vi "BX.Facade__LCR.vi"(0 "Data In":T11, 2 "Display State In":T2={"Orientation"=0, "ActivePicture"={"image type"=0, "image depth"=0, "image"=[], "mask"=[], "colors"=[], "Rectangle"={"left"=0, "top"=0, "right"=0, "bottom"=0}}, "Pictures"={"Normal"={"image type"=0, "image depth"=0, "image"=[], "mask"=[], "colors"=[], "Rectangle"={"left"=0, "top"=0, "right"=0, "bottom"=0}}, "Hilite"={"image type"=0, "image depth"=0, "image"=[], "mask"=[], "colors"=[], "Rectangle"={"left"=0, "top"=0, "right"=0, "bottom"=0}}}, "Text"={"String"="", "Font"={"Font Name:"="", "Size"=0, "Strikeout?"=FALSE, "Italic?"=FALSE, "Underline?"=FALSE, "Outline?"=FALSE, "Shadow?"=FALSE, "Bold?"=FALSE}, "TextColor"=0}, "RunTimeSettings"={"Highlight"=FALSE, "ShowButton"=FALSE, "Behaviour"=enum."Switch when pressed", "React if disabled"=FALSE, "Nudge Button"=TRUE, "ShowButton on Hover"=FALSE, "Button Type"=enum."System"}, "Messages"=[], "Status"=0, "XControl Label"="", "Boolean Value"=FALSE} {"Status" format="%.0x"}, 3 "Container State":T10) -> (6 "Data Out":T11, 7 "Display State Out":T2={"Orientation"=0, "ActivePicture"={"image type"=0, "image depth"=0, "image"=[], "mask"=[], "colors"=[], "Rectangle"={"left"=0, "top"=0, "right"=0, "bottom"=0}}, "Pictures"={"Normal"={"image type"=0, "image depth"=0, "image"=[], "mask"=[], "colors"=[], "Rectangle"={"left"=0, "top"=0, "right"=0, "bottom"=0}}, "Hilite"={"image type"=0, "image depth"=0, "image"=[], "mask"=[], "colors"=[], "Rectangle"={"left"=0, "top"=0, "right"=0, "bottom"=0}}}, "Text"={"String"="", "Font"={"Font Name:"="", "Size"=0, "Strikeout?"=FALSE, "Italic?"=FALSE, "Underline?"=FALSE, "Outline?"=FALSE, "Shadow?"=FALSE, "Bold?"=FALSE}, "TextColor"=0}, "RunTimeSettings"={"Highlight"=FALSE, "ShowButton"=FALSE, "Behaviour"=enum."Switch when pressed", "React if disabled"=FALSE, "Nudge Button"=TRUE, "ShowButton on Hover"=FALSE, "Button Type"=enum."System"}, "Messages"=[], "Status"=0, "XControl Label"="", "Boolean Value"=FALSE} {"Status" format="%.0x"}, 8 "Action":T1)   [LabVIEW 2011, in "BooleanXControl__LCR.xctl"]
doc: "Facade VI of the XControl"
uses:
  BooleanXControl__LCR.xctl
  BX.Data__LCR.ctl
  <vilib>/_xctls/Container State.ctl
  BX.State__LCR.ctl
  Controls/BX.Orientation__LCR.ctl
  <vilib>/picture/picture.llb/imagedata.ctl
  Controls/BX.RTSettings__LCR.ctl
  Controls/BX.Behaviour__LCR.ctl
  Controls/BX.ButtonType__LCR.ctl
  Controls/BX.Message__LCR.ctl
  Controls/BX.Commands__LCR.ctl
  <vilib>/_xctls/Action.ctl
  Controls/BX.Refs__LCR.ctl
  <userlib>/_OpenG.lib/file/file.llb/Strip Path Extension - Path__ogtk.vi
  <vilib>/Utility/inputDevices.llb/mouseAcquire.vi
  <vilib>/Utility/cursorutil.llb/Set Cursor (Icon Pict).vi
  <vilib>/_xctls/XControlSupport.lvlib
panel:
  in  "HiddenPath":path
  out "BooleanPicture":picture
  in  "ClassicButton":bool
  in  "ModernButton":bool
  out "BooleanString":string
  in  "SystemButton":bool
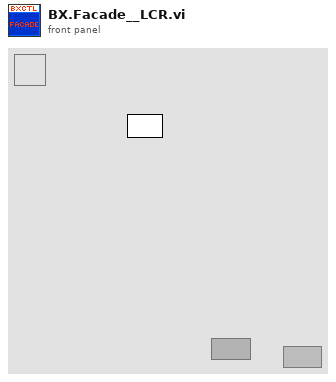
[diagram p1: front panel]
types:
  T1 = typedef "XControlSupport.lvlib/Action.ctl" = cluster{"Data Changed?":bool, "State Changed?":bool, "Action Name":string}
  T2 = typedef "BooleanXControl__LCR.xctl/BX.State__LCR.ctl" = cluster{"Orientation":T3, "ActivePicture":T4, "Pictures":cluster{"Normal":T4, "Hilite":T4}, "Text":cluster{"String":string, "Font":cluster{"Font Name:":string, "Size":i16, "Strikeout?":bool, "Italic?":bool, "Underline?":bool, "Outline?":bool, "Shadow?":bool, "Bold?":bool}, "TextColor":u32}, "RunTimeSettings":T5, "Messages":T8[], "Status":u16, "XControl Label":string, "Boolean Value":bool}
  T3 = typedef "BooleanXControl__LCR.xctl/BX.Orientation__LCR.ctl" = u8
  T4 = typedef "imagedata.ctl" = cluster{"image type":i32, "image depth":i32, "image":u8[], "mask":u8[], "colors":u32[], "Rectangle":cluster{"left":i16, "top":i16, "right":i16, "bottom":i16}}
  T5 = typedef "BooleanXControl__LCR.xctl/BX.RTSettings__LCR.ctl" = cluster{"Highlight":bool, "ShowButton":bool, "Behaviour":T6, "React if disabled":bool, "Nudge Button":bool, "ShowButton on Hover":bool, "Button Type":T7}
  T6 = typedef "BooleanXControl__LCR.xctl/BX.Behaviour__LCR.ctl" = enum16{"Switch when pressed", "Switch when released", "Switch until released"}
  T7 = typedef "BooleanXControl__LCR.xctl/BX.ButtonType__LCR.ctl" = enum16{"System", "Modern", "Classic", "Decoration"}
  T8 = typedef "BooleanXControl__LCR.xctl/BX.Message__LCR.ctl" = cluster{"Command":T9, "Parameter":variant}
  T9 = typedef "BooleanXControl__LCR.xctl/BX.Commands__LCR.ctl" = enum16{"None", "SetPicture", "SetFont", "SetText", "SetOrientation", "Redraw", "SetTextColor", "SetRTSettings", "MultipleUpdate", "RT.Button", "RT.Hilite", "RT.Behaviour", "RT.Disabled", "ShowGUI", "RT.Nudge", "RT.Hover", "RT.ButtonType"}
  T10 = typedef "XControlSupport.lvlib/Container State.ctl" = cluster{"Indicator?":bool, "Run Mode?":bool, " Refnum":refnum<vi>}
  T11 = typedef "BooleanXControl__LCR.xctl/BX.Data__LCR.ctl" = bool
  T12 = typedef "BooleanXControl__LCR.xctl/BX.Refs__LCR.ctl" = cluster{"HiddenPath":refnum<vi>, "String":refnum<vi>, "Picture":refnum<vi>, "XControl":refnum<vi>, "SystemButton":refnum<vi>, "ModernButton":refnum<vi>, "ClassicButton":refnum<vi>, "Decor Refnum":refnum<vi>}
  T13 = cluster{"button 1":bool, "button 2":bool, "button 3":bool, "button 4":bool}
  T14 = typedef "eventsource.ctl" = u32
  T15 = cluster{"Shift":bool, "Ctrl":bool, "Alt":bool, "Cmd":bool, "Opt":bool}
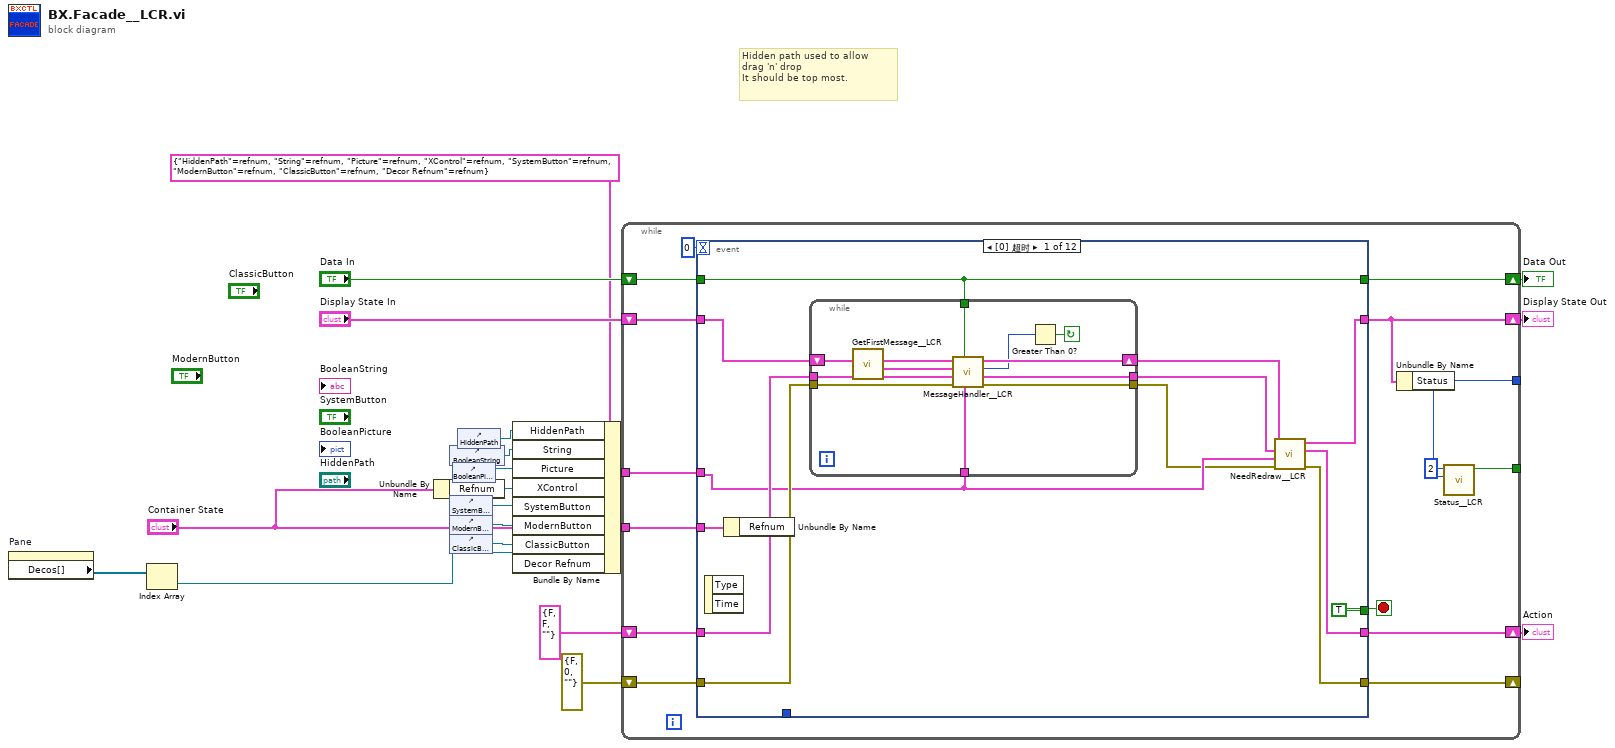
[diagram p0: block diagram]
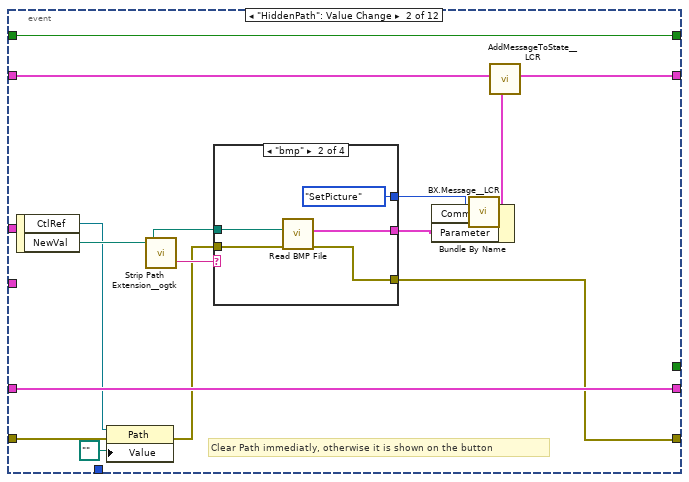
[diagram p2: hidden frame]
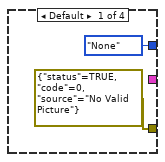
[diagram p3: hidden frame]
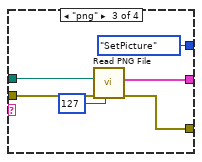
[diagram p4: hidden frame]
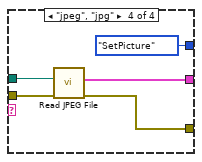
[diagram p5: hidden frame]
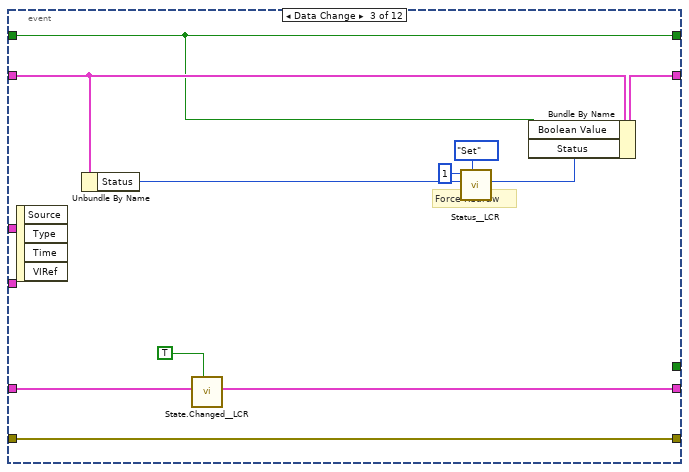
[diagram p6: hidden frame]
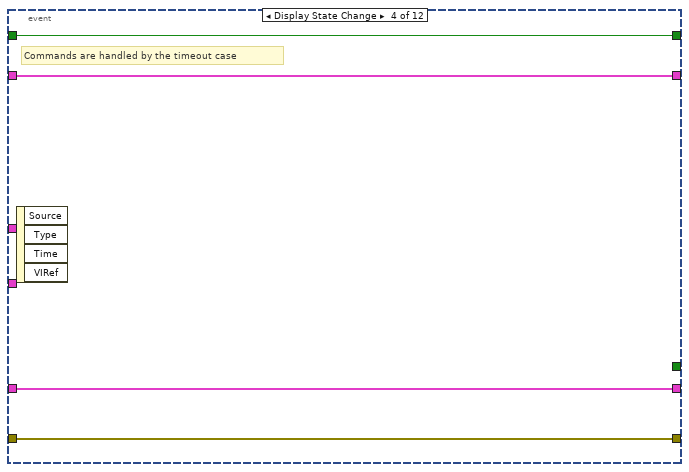
[diagram p7: hidden frame]
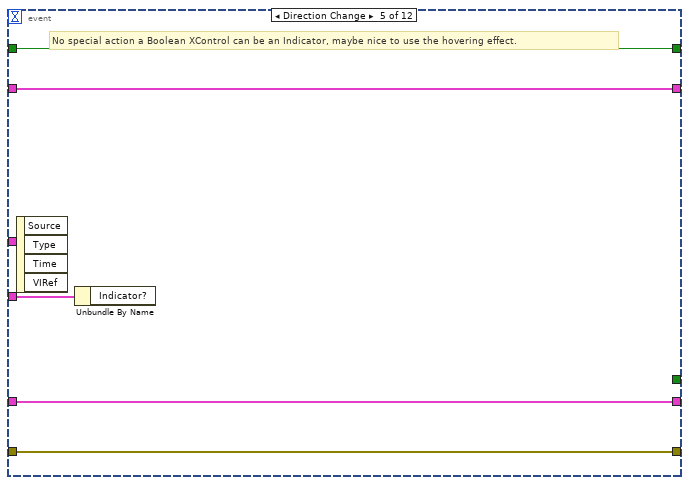
[diagram p8: hidden frame]
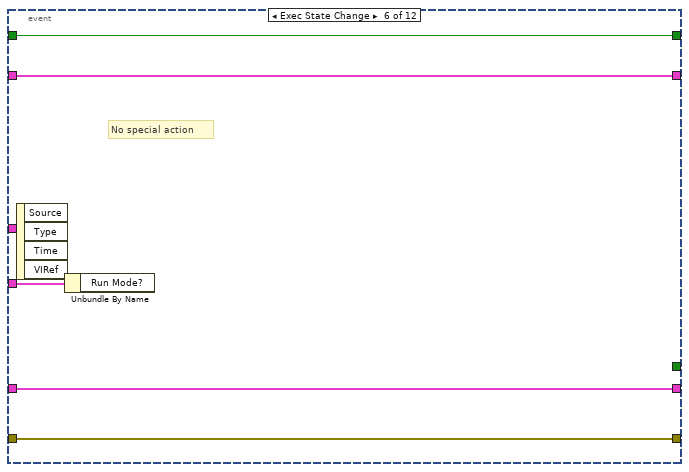
[diagram p9: hidden frame]
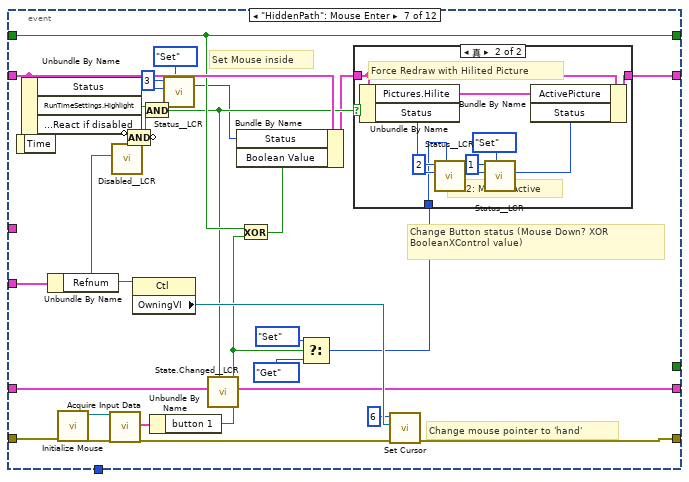
[diagram p10: hidden frame]
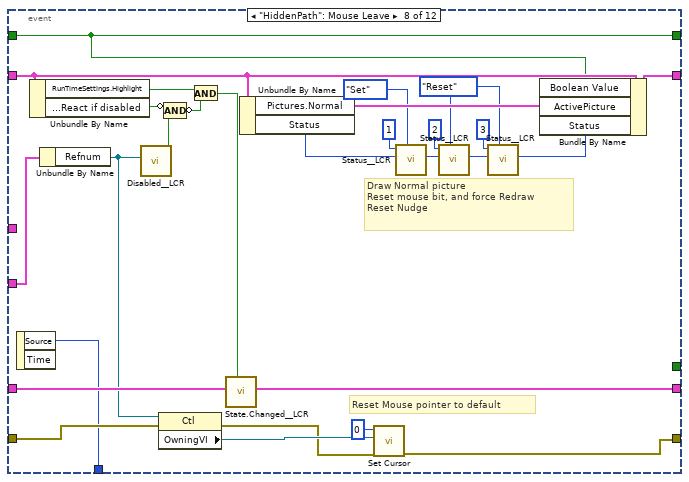
[diagram p12: hidden frame]
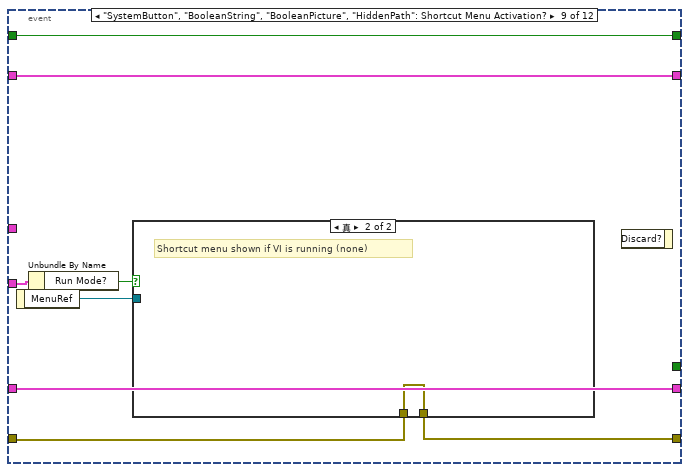
[diagram p13: hidden frame]
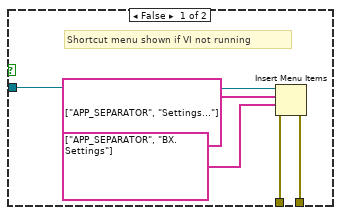
[diagram p14: hidden frame]
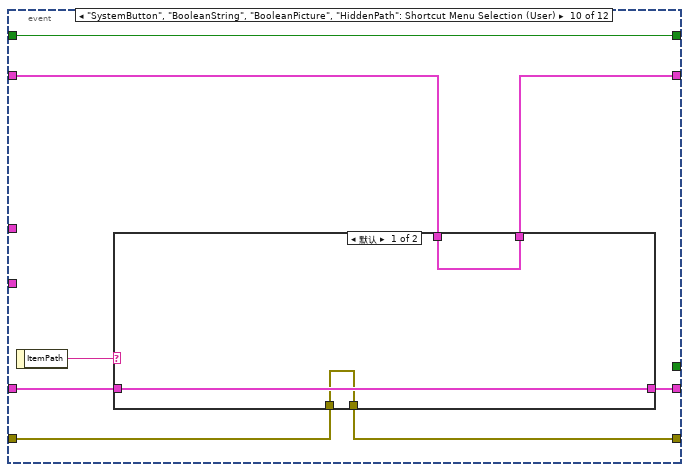
[diagram p15: hidden frame]
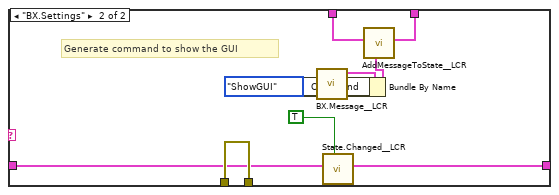
[diagram p16: hidden frame]
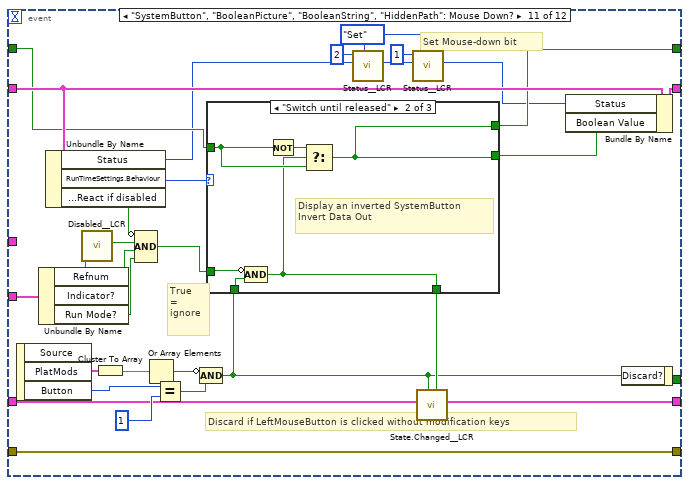
[diagram p17: hidden frame]
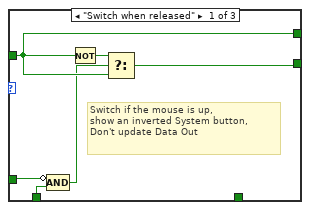
[diagram p18: hidden frame]
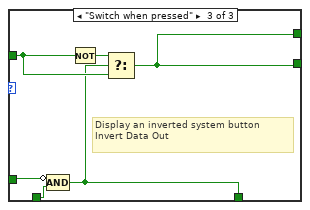
[diagram p19: hidden frame]
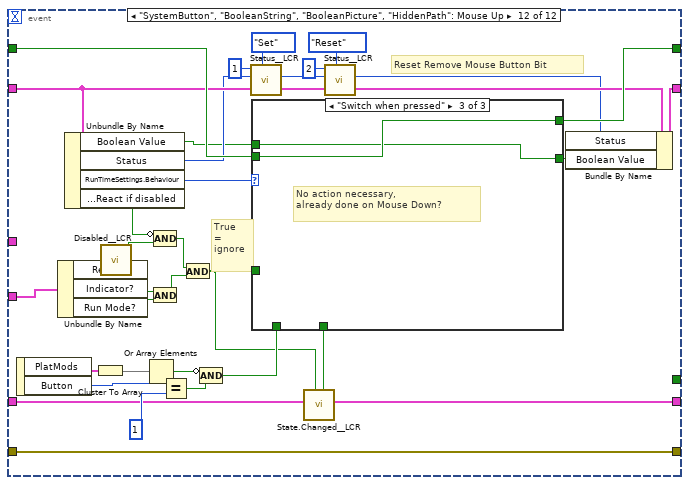
[diagram p20: hidden frame]
diagram:
  # "Hidden path used to allow\ndrag 'n' drop\nIt should be top most."
  n1 = property on="Pane" class="Pane"() -> ("Decos[]"=w2:refnum<vi>[])  [unwired: 2 in, 2 out]
  n2 = Index Array(array=w2) -> (element=w1:refnum<vi>)  [unwired: 1 in]
  n3 = Unbundle By Name("Container State") -> ("Refnum"=w7:refnum<vi>)
  n4 = control-ref of="BooleanString"() -> (w10:refnum<vi>)
  n5 = control-ref of="SystemButton"() -> (w6:refnum<vi>)
  n6 = control-ref of="ModernButton"() -> (w3:refnum<vi>)
  n7 = control-ref of="ClassicButton"() -> (w4:refnum<vi>)
  n8 = control-ref of="BooleanPicture"() -> (w9:refnum<vi>)
  n9 = control-ref of="HiddenPath"() -> (w11:refnum<vi>)
  n10 = Bundle By Name(cluster=T12 {"HiddenPath"=refnum, "String"=refnum, "Picture"=refnum, "XControl"=refnum, "SystemButton"=refnum, "ModernButton"=refnum, "ClassicButton"=refnum, "Decor Refnum"=refnum} ("BX.FP Refs"), "HiddenPath"=w11, "String"=w10, "Picture"=w9, "XControl"=w7, "SystemButton"=w6, "ModernButton"=w3, "ClassicButton"=w4, "Decor Refnum"=w1) -> (w5:T12)
  n11 = while {
    shift-right: [w23] -> w18
    shift-left: "Display State In" -> [w34]
    tunnel: "Container State" -> [w31]
    shift-right: [w29] -> w15
    shift-left: "Data In" -> [w30]
    shift-right: [w27] -> w17
    shift-left: T1 {"Data Changed?"=FALSE, "State Changed?"=FALSE, "Action Name"=""} ("Action") -> [w28]
    shift-right: [w25] -> _
    shift-left: errorcluster {"status"=FALSE, "code"=0, "source"=""} ("error in (no error)") -> [w26]
    tunnel: w5 -> [w24]
    tunnel: [w21] -> _
    tunnel: [w20] -> _
    stop <- w33 stop-if-true
    n12 = event shown="[0] 超时" {
      selector: _ -> [_ _ _ _ _ _ _ _ _ _ _ _]
      dyn-events: _ -> [_ _ _ _ _ _ _ _ _ _ _ _]
      timeout: 0 -> [_ _ _ _ _ _ _ _ _ _ _ _]
      tunnel: w34 -> [w42 w62 w103 w104 w111 w114 w146 w185 w189 w202 w244 w287]
      tunnel: [w43 w60 w102 w104 w111 w114 w145 w184 w189 w201 w234 w280] -> w23
      tunnel: [TRUE _ _ _ _ _ _ _ _ _ _ _] -> w33
      tunnel: w31 -> [w46 _ _ _ w112 w117 w141 w180 w193 _ w243 w286]
      tunnel: w30 -> [w41 w74 w98 w107 w110 w116 w130 w160 w191 w205 w228 w299]
      tunnel: [w41 w74 w98 w107 w110 w116 w130 w160 w191 w205 w241 w298] -> w29
      tunnel: [w45 w73 w100 w105 w109 w115 w136 w181 w190 w207 w235 w281] -> w27
      tunnel: w28 -> [w39 w73 w101 w105 w109 w115 w137 w182 w190 w206 w236 w282]
      tunnel: w26 -> [w40 w66 w99 w106 w108 w113 w131 w173 w188 w204 w232 w278]
      tunnel: [w44 w64 w99 w106 w108 w113 w129 w171 w187 w203 w232 w278] -> w25
      tunnel: w24 -> [w36 _ _ _ _ _ _ _ _ _ _ _]
      tunnel: [_ _ _ _ _ _ _ w159 _ _ _ _] -> _
      event Timeout {
        n13 = event-data() -> ()  [unwired: 1 in, 2 out]
        n14 = Unbundle By Name(w46) -> ()  [unwired: 1 out]
        n15 = while {
          shift-right: [w58] -> w37
          shift-left: w42 -> [w50]
          tunnel: w41 -> [w59]
          tunnel: w36 -> [w57]
          tunnel: w40 -> [w56]
          tunnel: w39 -> [w55]
          tunnel: [w54] -> w38
          tunnel: [w53] -> w35
          stop <- w51 continue-if-true
          n16 = call "GetFirstMessage__LCR.vi"("State In"=w50) -> ("State Out"=w49:T2, "Message"=w48:T8)  [unwired: 9 in]
          n17 = call "MessageHandler__LCR.vi"("reference"=w57, "Data In"=w59, "error in (no error)"=w56, "Action In"=w55, "Message"=w48, "State In"=w49) -> ("error out"=w53:errorcluster, "Action Out"=w54:T1, "Remaining"=w52:i32, "State Out"=w58:T2)  [unwired: 2 in]
          n18 = Greater Than 0?(x=w52) -> (x > 0?=w51:bool)
        }
        n19 = call "NeedRedraw__LCR.vi"("error in (no error)"=w35, "BX.FP Refs"=w36, "Action In"=w38, "Display State In"=w37) -> ("error out"=w44:errorcluster, "Action Out"=w45:T1, "Display State Out"=w43:T2)  [unwired: 5 in]
      }
      event "HiddenPath": Value Change {
        # "Clear Path immediatly, otherwise it is shown on the button"
        n20 = event-data() -> ("CtlRef"=w67:refnum<vi>, "NewVal"=w71:path)  [unwired: 1 in]
        n21 = property class="Path"(reference=w67, error in=w66, "Value"=path "") -> (error out=w65:errorcluster)  [unwired: 1 out]
        n22 = call-poly <userlib>:"Strip Path Extension__ogtk.vi"("path"=w71) -> ("extension"=w72:string)  [unwired: 1 out]
        n23 = case shown="\"bmp\"" w72 {
          tunnel: w71 -> [_ w81 w87 w92]
          tunnel: [errorcluster {"status"=TRUE, "code"=0, "source"="No Valid Picture"} ("error out") w80 w86 w91] -> w64
          tunnel: [_ w79 w85 w90] -> w69
          tunnel: w65 -> [_ w78 w83 w89]
          tunnel: [BX.Commands__LCR."None" ("Command") BX.Commands__LCR."SetPicture" ("Command") BX.Commands__LCR."SetPicture" ("Command") BX.Commands__LCR."SetPicture" ("Command")] -> w63
          frame Default {
          }
          frame "bmp" {
            n24 = call <vilib>:"Read BMP File.vi"("error in (no error)"=w78, "path to BMP file"=w81) -> ("error out"=w80:errorcluster, "image data"=w79:T4)  [unwired: 7 in, 1 out]
          }
          frame "png" {
            n25 = call <vilib>:"Read PNG File.vi"("Transparency Thresh"=u8 127, "error in (no error)"=w83, "path to PNG file"=w87) -> ("error out"=w86:errorcluster, "image data"=w85:T4)  [unwired: 6 in, 1 out]
          }
          frame "jpeg", "jpg" {
            n26 = call <vilib>:"Read JPEG File.vi"("error in (no error)"=w89, "path to JPEG file"=w92) -> ("error out"=w91:errorcluster, "image data"=w90:T4)  [unwired: 7 in, 1 out]
          }
        }
        n27 = call "BX.Message__LCR.vi"() -> ("Messages"=w70:T8)  [unwired: 11 in]
        n28 = Bundle By Name(cluster=w70, "Command"=w63, "Parameter"=w69) -> (w61:T8)
        n29 = call "AddMessageToState__LCR.vi"("Message"=w61, "State In"=w62) -> ("State Out"=w60:T2)  [unwired: 9 in]
      }
      event Data Change {
        # "Force Redraw"
        n30 = event-data() -> ()  [unwired: 1 in, 4 out]
        n31 = Unbundle By Name(w103) -> ("Status"=w97:u16)
        n32 = call "State.Changed__LCR.vi"("State Changed?"=TRUE, "Action in"=w101) -> ("Action"=w100:T1)  [unwired: 9 in]
        n33 = call "Status__LCR.vi"("Action (Get)"=enum16{"Get", "Set", "Reset"}."Set", "Status In"=w97, "Bit"=u16 1) -> ("Status Out"=w94:u16)  [unwired: 7 in, 1 out]
        n34 = Bundle By Name(cluster=w103, "Boolean Value"=w98, "Status"=w94) -> (w102:T2)
      }
      event Display State Change {
        # "Commands are handled by the timeout case"
        n35 = event-data() -> ()  [unwired: 1 in, 4 out]
      }
      event Direction Change {
        # "No special action a Boolean XControl can be an Indicator, maybe nice to use the hovering effect."
        n36 = event-data() -> ()  [unwired: 1 in, 4 out]
        n37 = Unbundle By Name(w112) -> ()  [unwired: 1 out]
      }
      event Exec State Change {
        # "No special action"
        n38 = event-data() -> ()  [unwired: 1 in, 4 out]
        n39 = Unbundle By Name(w117) -> ()  [unwired: 1 out]
      }
      event "HiddenPath": Mouse Enter {
        # "Set Mouse inside"
        # "Change Button status (Mouse Down? XOR  \nBooleanXControl value)"
        # "Change mouse pointer to 'hand'"
        n40 = event-data() -> ()  [unwired: 1 in, 1 out]
        n41 = Unbundle By Name(w146) -> ("Status"=w122:u16, "RunTimeSettings.Highlight"=w147:bool, "RunTimeSettings.React if disabled"=w134:bool)
        n42 = Unbundle By Name(w141) -> ("Refnum"=w135:refnum<vi>)
        n43 = call <vilib>:"Initialize Mouse.vi"("error in (no error)"=w131) -> ("error out"=w144:errorcluster, "device ID"=w143:refnum<k1>)  [unwired: 9 in]
        n44 = call-poly <vilib>:"Acquire Input Data.vi"("device ID"=w143, "error in (no error)"=w144) -> ("button info"=w142:T13, "error out"=w139:errorcluster)  [unwired: 14 in, 2 out]
        n45 = call "Disabled__LCR.vi"("Control"=w135) -> ("Disabled?"=w133:bool)  [unwired: 10 in]
        n46 = Compound Arithmetic op=AND(invert w134, w133) -> (invert w132:bool)
        n47 = property class="Ctl"(reference=w135) -> ("OwningVI"=w140:refnum<vi>)  [unwired: 1 in, 2 out]
        n48 = And(x=w147, y=w132) -> (x .and. y?=w124:bool)
        n49 = Unbundle By Name(w142) -> ("button 1"=w126:bool)
        n50 = call "Status__LCR.vi"("Action (Get)"=enum16{"Get", "Set", "Reset"}."Set", "Status In"=w122, "Bit"=u16 3) -> ("Status Out"=w119:u16)  [unwired: 7 in, 1 out]
        n51 = call "State.Changed__LCR.vi"("State Changed?"=w124, "Action in"=w137) -> ("Action"=w136:T1)  [unwired: 9 in]
        n52 = Exclusive Or(1:w126, 2:w130) -> (0:w118:T11)
        n53 = Bundle By Name(cluster=w146, "Status"=w119, "Boolean Value"=w118) -> (w120:T2)
        n54 = Select(t=enum16{"Get", "Set", "Reset"}."Set" ("Action (Get)"), s=w126, f=enum16{"Get", "Set", "Reset"}."Get" ("Action (Get)")) -> (s? t:f=w125:enum16{"Get", "Set", "Reset"})
        n55 = case shown="真" w124 {
          tunnel: w120 -> [w148 w158]
          tunnel: [w148 w157] -> w145
          tunnel: w125 -> [_ w153]
          frame False {
            # "Don't change picture if Hilite is False OR (control is disabled\nAND shouldn't react if disabled)"
          }
          frame True {
            # "Force Redraw with Hilited Picture"
            # "Bit 2: Mouse Active"
            n56 = Unbundle By Name(w158) -> ("Pictures.Hilite"=w156:T4, "Status"=w155:u16)
            n57 = call "Status__LCR.vi"("Action (Get)"=w153, "Status In"=w155, "Bit"=u16 2) -> ("Status Out"=w152:u16)  [unwired: 7 in, 1 out]
            n58 = call "Status__LCR.vi"("Action (Get)"=enum16{"Get", "Set", "Reset"}."Set", "Status In"=w152, "Bit"=u16 1) -> ("Status Out"=w150:u16)  [unwired: 7 in, 1 out]
            n59 = Bundle By Name(cluster=w158, "ActivePicture"=w156, "Status"=w150) -> (w157:T2)
          }
        }
        n60 = call-poly <vilib>:"Set Cursor.vi"("error in (no error)"=w139, "VI reference (current VI)"=w140, "icon"=u16 6) -> ("error out"=w129:errorcluster)  [unwired: 7 in, 1 out]
      }
      event "HiddenPath": Mouse Leave {
        w162 = enum16{"Get", "Set", "Reset"}."Reset" ("Action (Get)")
        # "Draw Normal picture\nReset mouse bit, and force Redraw\nReset Nudge"
        # "Reset Mouse pointer to default"
        n61 = event-data() -> ("Source"=w159:T14)  [unwired: 1 in, 1 out]
        n62 = Unbundle By Name(w185) -> ("RunTimeSettings.Highlight"=w186:bool, "RunTimeSettings.React if disabled"=w179:bool)
        n63 = Unbundle By Name(w180) -> ("Refnum"=w175:refnum<vi>)
        n64 = call "Disabled__LCR.vi"("Control"=w175) -> ("Disabled?"=w178:bool)  [unwired: 10 in]
        n65 = property class="Ctl"(reference=w175, error in=w173) -> (error out=w172:errorcluster, "OwningVI"=w174:refnum<vi>)  [unwired: 1 out]
        n66 = Compound Arithmetic op=AND(invert w179, w178) -> (invert w177:bool)
        n67 = And(x=w186, y=w177) -> (x .and. y?=w183:bool)
        n68 = call "State.Changed__LCR.vi"("State Changed?"=w183, "Action in"=w182) -> ("Action"=w181:T1)  [unwired: 9 in]
        n69 = Unbundle By Name(w185) -> ("Pictures.Normal"=w170:T4, "Status"=w168:u16)
        n70 = call-poly <vilib>:"Set Cursor.vi"("error in (no error)"=w172, "VI reference (current VI)"=w174, "icon"=u16 0) -> ("error out"=w171:errorcluster)  [unwired: 7 in, 1 out]
        n71 = call "Status__LCR.vi"("Action (Get)"=enum16{"Get", "Set", "Reset"}."Set", "Status In"=w168, "Bit"=u16 1) -> ("Status Out"=w166:u16)  [unwired: 7 in, 1 out]
        n72 = call "Status__LCR.vi"("Action (Get)"=w162, "Status In"=w166, "Bit"=u16 2) -> ("Status Out"=w164:u16)  [unwired: 7 in, 1 out]
        n73 = call "Status__LCR.vi"("Action (Get)"=w162, "Status In"=w164, "Bit"=u16 3) -> ("Status Out"=w163:u16)  [unwired: 7 in, 1 out]
        n74 = Bundle By Name(cluster=w185, "Boolean Value"=w160, "ActivePicture"=w170, "Status"=w163) -> (w184:T2)
      }
      event "SystemButton", "BooleanString", "BooleanPicture", "HiddenPath": Shortcut Menu Activation? {
        n75 = event-data() -> ("MenuRef"=w194:refnum<k9>)  [unwired: 1 in]
        n76 = Unbundle By Name(w193) -> ("Run Mode?"=w192:bool)
        n77 = case shown="真" w192 {
          tunnel: w194 -> [w199 _]
          tunnel: w188 -> [w196 w200]
          tunnel: [w195 w200] -> w187
          frame False {
            # "Shortcut menu shown if VI not running"
            n78 = Insert Menu Items(6:w196, 7:string[] ["APP_SEPARATOR", "BX.Settings"] ("item tags"), 8:string[] ["APP_SEPARATOR", "Settings..."] ("item names"), 9:w199) -> (0:w195:errorcluster)  [unwired: 2 in, 2 out]
          }
          frame True {
            # "Shortcut menu shown if VI is running (none)"
          }
        }
        n79 = event-data() -> ()  [unwired: 2 in, 1 out]
      }
      event "SystemButton", "BooleanString", "BooleanPicture", "HiddenPath": Shortcut Menu Selection (User) {
        n80 = event-data() -> ("ItemPath"=w208:string)  [unwired: 1 in]
        n81 = case shown="默认" w208 {
          tunnel: [w211 w212] -> w207
          tunnel: w206 -> [w211 w214]
          tunnel: w204 -> [w210 w215]
          tunnel: [w210 w215] -> w203
          tunnel: w202 -> [w209 w218]
          tunnel: [w209 w217] -> w201
          frame Default {
          }
          frame "BX.Settings" {
            # "Generate command to show the GUI"
            n82 = call "BX.Message__LCR.vi"() -> ("Messages"=w220:T8)  [unwired: 11 in]
            n83 = Bundle By Name(cluster=w220, "Command"=BX.Commands__LCR."ShowGUI") -> (w216:T8)
            n84 = call "State.Changed__LCR.vi"("State Changed?"=TRUE, "Action in"=w214) -> ("Action"=w212:T1)  [unwired: 9 in]
            n85 = call "AddMessageToState__LCR.vi"("Message"=w216, "State In"=w218) -> ("State Out"=w217:T2)  [unwired: 9 in]
          }
        }
      }
      event "SystemButton", "BooleanPicture", "BooleanString", "HiddenPath": Mouse Down? {
        w223 = enum16{"Get", "Set", "Reset"}."Set" ("Action (Get)")
        # "Set Mouse-down bit"
        # "True\n= \nignore"
        # "Discard if LeftMouseButton is clicked without modification keys"
        n86 = event-data() -> ("PlatMods"=w250:T15, "Button"=w245:u16)  [unwired: 1 in, 1 out]
        n87 = Unbundle By Name(w243) -> ("Refnum"=w240:refnum<vi>, "Indicator?"=w231:bool, "Run Mode?"=w230:bool)
        n88 = Unbundle By Name(w244) -> ("Status"=w226:u16, "RunTimeSettings.Behaviour"=w242:T6, "RunTimeSettings.React if disabled"=w239:bool)
        n89 = call "Disabled__LCR.vi"("Control"=w240) -> ("Disabled?"=w238:bool)  [unwired: 10 in]
        n90 = Cluster To Array(cluster=w250) -> (array=w249:bool[])
        n91 = Compound Arithmetic op=AND(invert w239, w238, w231, w230) -> (w229:bool)
        n92 = Or Array Elements(Boolean array=w249) -> (logical OR=w248:bool)
        n93 = Equal?(x=w245, y=u16 1 ("x")) -> (x = y?=w246:bool)
        n94 = Compound Arithmetic op=AND(invert w248, w246) -> (w233:bool)
        n95 = case shown="\"Switch until released\"" w242 {
          tunnel: w228 -> [w254 w261 w267]
          tunnel: [w255 w258 w264] -> w221
          tunnel: w233 -> [w252 w259 w265]
          tunnel: [w254 w258 w264] -> w241
          tunnel: w229 -> [w253 w260 w266]
          tunnel: [_ w257 w263] -> w237
          frame "Switch when released" {
            # "Switch if the mouse is up,\nshow an inverted System button,\nDon't update Data Out"
            n96 = Compound Arithmetic op=AND(invert w253, w252) -> (w251:bool)
            n97 = Not(x=w254) -> (.not. x?=w256:T11)
            n98 = Select(t=w256, s=w251, f=w254) -> (s? t:f=w255:T11)
          }
          frame "Switch until released" {
            # "Display an inverted SystemButton\nInvert Data Out"
            n99 = Compound Arithmetic op=AND(invert w260, w259) -> (w257:bool)
            n100 = Not(x=w261) -> (.not. x?=w262:T11)
            n101 = Select(t=w262, s=w257, f=w261) -> (s? t:f=w258:T11)
          }
          frame "Switch when pressed" {
            # "Display an inverted system button\nInvert Data Out"
            n102 = Compound Arithmetic op=AND(invert w266, w265) -> (w263:bool)
            n103 = Not(x=w267) -> (.not. x?=w268:T11)
            n104 = Select(t=w268, s=w263, f=w267) -> (s? t:f=w264:T11)
          }
        }
        n105 = call "Status__LCR.vi"("Action (Get)"=w223, "Status In"=w226, "Bit"=u16 2) -> ("Status Out"=w225:u16)  [unwired: 7 in, 1 out]
        n106 = call "Status__LCR.vi"("Action (Get)"=w223, "Status In"=w225, "Bit"=u16 1) -> ("Status Out"=w224:u16)  [unwired: 7 in, 1 out]
        n107 = call "State.Changed__LCR.vi"("Data Changed?"=w237, "State Changed?"=w233, "Action in"=w236) -> ("Action"=w235:T1)  [unwired: 8 in]
        n108 = Bundle By Name(cluster=w244, "Status"=w224, "Boolean Value"=w221) -> (w234:T2)
        n109 = event-data("Discard?"=w233) -> ()  [unwired: 1 in, 1 out]
      }
      event "SystemButton", "BooleanString", "BooleanPicture", "HiddenPath": Mouse Up {
        # "Reset Remove Mouse Button Bit"
        # "True\n= \nignore"
        n110 = event-data() -> ("PlatMods"=w296:T15, "Button"=w297:u16)  [unwired: 1 in]
        n111 = Unbundle By Name(w286) -> ("Refnum"=w294:refnum<vi>, "Indicator?"=w290:bool, "Run Mode?"=w291:bool)
        n112 = Unbundle By Name(w287) -> ("Boolean Value"=w269:bool, "Status"=w273:u16, "RunTimeSettings.Behaviour"=w285:T6, "RunTimeSettings.React if disabled"=w293:bool)
        n113 = Cluster To Array(cluster=w296) -> (array=w302:bool[])
        n114 = call "Disabled__LCR.vi"("Control"=w294) -> ("Disabled?"=w292:bool)  [unwired: 10 in]
        n115 = Or Array Elements(Boolean array=w302) -> (logical OR=w301:bool)
        n116 = And(x=w290, y=w291) -> (x .and. y?=w289:bool)
        n117 = Compound Arithmetic op=AND(invert w293, w292) -> (w288:bool)
        n118 = Equal?(x=w297, y=u16 1 ("x")) -> (x = y?=w300:bool)
        n119 = And(x=w288, y=w289) -> (x .and. y?=w279:bool)
        n120 = Compound Arithmetic op=AND(invert w301, w300) -> (w284:bool)
        n121 = call "Status__LCR.vi"("Action (Get)"=enum16{"Get", "Set", "Reset"}."Set", "Status In"=w273, "Bit"=u16 1) -> ("Status Out"=w274:u16)  [unwired: 7 in, 1 out]
        n122 = case shown="\"Switch when pressed\"" w285 {
          tunnel: w299 -> [w307 w313 w316]
          tunnel: [w303 w309 w316] -> w298
          tunnel: [w304 w310 _] -> w283
          tunnel: w279 -> [w306 w312 _]
          tunnel: w284 -> [w305 w311 _]
          tunnel: [w303 w309 w315] -> w270
          tunnel: w269 -> [_ _ w315]
          frame "Switch when released" {
            # "Invert DATA Out, \nset System Button\nto the same state \n(should already be there)"
            n123 = Not(x=w307) -> (.not. x?=w308:T11)
            n124 = Compound Arithmetic op=AND(invert w306, w305) -> (w304:bool)
            n125 = Select(t=w308, s=w304, f=w307) -> (s? t:f=w303:T11)
            n126 = local write "ModernButton"(w303) -> ()
            n127 = local write "SystemButton"(w303) -> ()
            n128 = local write "ClassicButton"(w303) -> ()
          }
          frame "Switch until released" {
            # "Invert Data Out and set SystemButton\nto the same state"
            n129 = Not(x=w313) -> (.not. x?=w314:T11)
            n130 = Compound Arithmetic op=AND(invert w312, w311) -> (w310:bool)
            n131 = Select(t=w314, s=w310, f=w313) -> (s? t:f=w309:T11)
            n132 = local write "ModernButton"(w309) -> ()
            n133 = local write "SystemButton"(w309) -> ()
            n134 = local write "ClassicButton"(w309) -> ()
          }
          frame "Switch when pressed" {
            # "No action necessary, \nalready done on Mouse Down?"
          }
        }
        n135 = call "State.Changed__LCR.vi"("Data Changed?"=w283, "State Changed?"=w279, "Action in"=w282) -> ("Action"=w281:T1)  [unwired: 8 in]
        n136 = call "Status__LCR.vi"("Action (Get)"=enum16{"Get", "Set", "Reset"}."Reset", "Status In"=w274, "Bit"=u16 2) -> ("Status Out"=w277:u16)  [unwired: 7 in, 1 out]
        n137 = Bundle By Name(cluster=w287, "Status"=w277, "Boolean Value"=w270) -> (w280:T2)
      }
    }
    n138 = Unbundle By Name(w23) -> ("Status"=w21:u16)
    n139 = call "Status__LCR.vi"("Status In"=w21, "Bit"=u16 2) -> ("Bit Value Out"=w20:bool)  [unwired: 8 in, 1 out]
  }
  "Display State Out" <- w18
  "Data Out" <- w15
  "Action" <- w17
